vi "OFFSETEXPAND.vi"(9 "address string":string) -> ()   [LabVIEW 2013]
panel:
  out "data":string
  out "Expand":dbl format="%.2f"
  out "offset":dbl format="%.2f"
  out "data 2":string
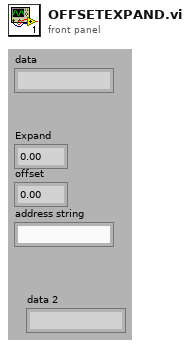
[diagram p1: front panel]
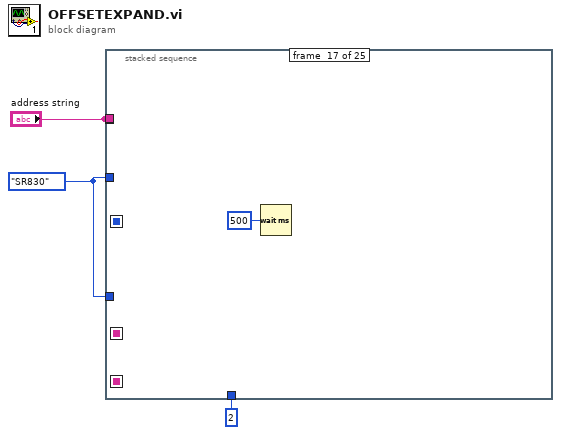
[diagram p0: block diagram]
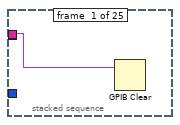
[diagram p2: hidden frame]
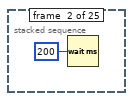
[diagram p3: hidden frame]
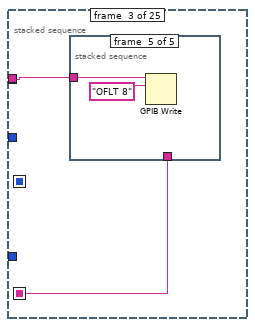
[diagram p4: hidden frame]
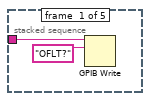
[diagram p5: hidden frame]
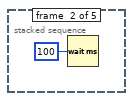
[diagram p6: hidden frame]
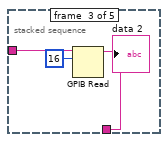
[diagram p7: hidden frame]
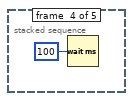
[diagram p8: hidden frame]
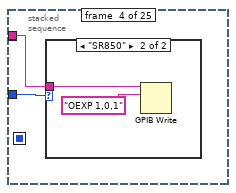
[diagram p9: hidden frame]
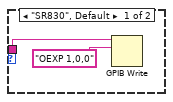
[diagram p10: hidden frame]
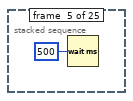
[diagram p11: hidden frame]
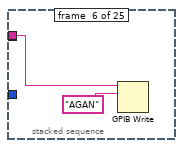
[diagram p12: hidden frame]
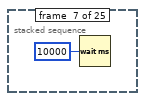
[diagram p13: hidden frame]
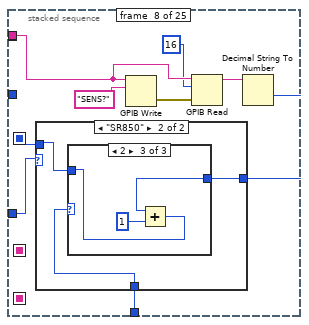
[diagram p14: hidden frame]
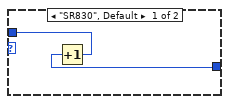
[diagram p15: hidden frame]
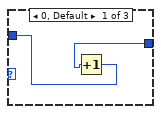
[diagram p16: hidden frame]
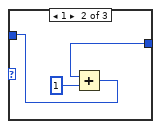
[diagram p17: hidden frame]
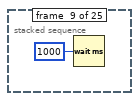
[diagram p18: hidden frame]
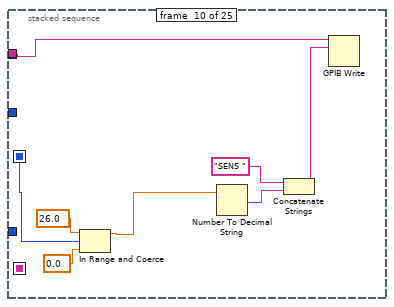
[diagram p19: hidden frame]
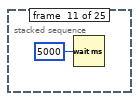
[diagram p20: hidden frame]
diagram:
  w2 = enum16{"SR830", "SR850"}."SR830" ("Lockin Type")
  n1 = stacked-sequence {
    seq-local: [_ _ _ _ _ _ _ _ _ _ _ _ _ _ _ _ _ w67 _ _ _ _ _ _ _] -> [_ _ _ _ _ _ _ _ _ _ _ _ _ _ _ _ _ _ _ w79 _ _ _ _ _]
    seq-local: [_ _ _ _ _ _ _ w29 _ _ _ _ _ _ _ _ _ _ _ _ _ _ _ _ _] -> [_ _ _ _ _ _ _ _ _ w51 _ _ _ _ _ _ _ _ _ _ _ _ _ _ _]
    seq-local: [_ _ w6 _ _ _ _ _ _ _ _ _ _ _ _ _ _ _ _ _ _ _ _ _ _] -> [_ _ _ _ _ _ _ _ _ _ _ _ _ _ _ _ _ _ _ _ _ _ _ w98 w104]
    tunnel: "address string" -> [w4 _ w7 _ _ _ _ w33 _ w57 _ w60 _ w62 _ w64 _ w72 _ w81 _ w94 _ w99 _]
    tunnel: "address string" -> [_ _ _ w18 _ w25 _ _ _ _ _ _ _ _ _ _ _ _ _ _ _ _ _ _ _]
    tunnel: w2 -> [_ _ _ _ _ _ _ w27 _ _ _ _ _ _ _ _ _ _ _ w76 _ _ _ _ _]
    tunnel: w2 -> [_ _ _ w17 _ _ _ _ _ _ _ _ _ _ _ _ _ _ _ _ _ _ _ _ _]
    tunnel: u16 2 ("Expand by") -> [_ _ _ _ _ _ _ w28 _ _ _ _ _ _ _ _ _ _ _ w75 _ _ _ _ _]
    frame #0 {
      n2 = GPIB Clear(3:w4) -> ()  [unwired: 1 in, 2 out]
    }
    frame #1 {
      n3 = Wait (ms)(milliseconds to wait=u32 200) -> ()  [unwired: 1 out]
    }
    frame #2 {
      n4 = stacked-sequence {
        tunnel: w7 -> [w9 _ w13 _ w16]
        tunnel: [_ _ w11 _ _] -> w6
        frame #0 {
          n5 = GPIB Write(0:w9, 1:"OFLT?" ("data")) -> ()  [unwired: 3 in, 2 out]
        }
        frame #1 {
          n6 = Wait (ms)(milliseconds to wait=u32 100) -> ()  [unwired: 1 out]
        }
        frame #2 {
          n7 = GPIB Read(0:w13, 1:16 ("byte count")) -> (5:w11:string)  [unwired: 3 in, 2 out]
          "data 2" <- w11
        }
        frame #3 {
          n8 = Wait (ms)(milliseconds to wait=u32 100) -> ()  [unwired: 1 out]
        }
        frame #4 {
          n9 = GPIB Write(0:w16, 1:"OFLT 8" ("data")) -> ()  [unwired: 3 in, 2 out]
        }
      }
    }
    frame #3 {
      n10 = case shown="\"SR850\"" w17 {
        tunnel: w18 -> [w19 w22]
        frame "SR830", Default {
          n11 = GPIB Write(0:w19, 1:"OEXP 1,0,0" ("data")) -> ()  [unwired: 3 in, 2 out]
        }
        frame "SR850" {
          n12 = GPIB Write(0:w22, 1:"OEXP 1,0,1" ("data")) -> ()  [unwired: 3 in, 2 out]
        }
      }
    }
    frame #4 {
      n13 = Wait (ms)(milliseconds to wait=u32 500) -> ()  [unwired: 1 out]
    }
    frame #5 {
      n14 = GPIB Write(0:w25, 1:"AGAN" ("data")) -> ()  [unwired: 3 in, 2 out]
    }
    frame #6 {
      n15 = Wait (ms)(milliseconds to wait=u32 10000) -> ()  [unwired: 1 out]
    }
    frame #7 {
      n16 = GPIB Write(0:w33, 1:"SENS?" ("data")) -> (6:w34:errorcluster)  [unwired: 3 in, 1 out]
      n17 = GPIB Read(0:w33, 1:16 ("byte count"), 3:w34) -> (5:w31:string)  [unwired: 2 in, 2 out]
      n18 = Decimal String To Number(string=w31) -> (number=w30:i32)  [unwired: 2 in, 1 out]
      n19 = case shown="\"SR850\"" w27 {
        tunnel: w30 -> [w37 w39]
        tunnel: [w36 w38] -> w29
        tunnel: w28 -> [_ w40]
        frame "SR830", Default {
          n20 = Increment(x=w37) -> (x+1=w36:i32)
        }
        frame "SR850" {
          n21 = case shown="2" w40 {
            tunnel: w39 -> [w42 w45 w48]
            tunnel: [w41 w43 w46] -> w38
            frame 0, Default {
              n22 = Increment(x=w42) -> (x+1=w41:i32)
            }
            frame 1 {
              n23 = Add(x=w45, y=1) -> (x+y=w43:i32)
            }
            frame 2 {
              n24 = Add(x=w48, y=1) -> (x+y=w46:i32)
            }
          }
        }
      }
    }
    frame #8 {
      n25 = Wait (ms)(milliseconds to wait=u32 1000) -> ()  [unwired: 1 out]
    }
    frame #9 {
      n26 = In Range and Coerce(upper limit=26.0, x=w51, lower limit=0.0) -> (coerced(x)=w50:dbl)  [unwired: 1 out]
      n27 = Number To Decimal String(number=w50) -> (decimal integer string=w56:string)  [unwired: 1 in]
      n28 = Concatenate Strings("SENS " ("string"), w56) -> (w54:string)
      n29 = GPIB Write(0:w57, 1:w54) -> ()  [unwired: 3 in, 2 out]
    }
    frame #10 {
      n30 = Wait (ms)(milliseconds to wait=u32 5000) -> ()  [unwired: 1 out]
    }
    frame #11 {
      n31 = GPIB Write(0:w60, 1:"AOFF 1" ("data")) -> ()  [unwired: 3 in, 2 out]
    }
    frame #12 {
      n32 = Wait (ms)(milliseconds to wait=u32 1000) -> ()  [unwired: 1 out]
    }
    frame #13 {
      n33 = GPIB Clear(3:w62) -> ()  [unwired: 1 in, 2 out]
    }
    frame #14 {
      n34 = Wait (ms)(milliseconds to wait=u32 500) -> ()  [unwired: 1 out]
    }
    frame #15 {
      n35 = GPIB Write(0:w64, 1:"OEXP? 1" ("data")) -> ()  [unwired: 3 in, 2 out]
    }
    frame #16 {
      n36 = Wait (ms)(milliseconds to wait=u32 500) -> ()  [unwired: 1 out]
    }
    frame #17 {
      n37 = GPIB Read(0:w72, 1:512 ("byte count")) -> (5:w69:string)  [unwired: 3 in, 2 out]
      "data" <- w69
      n38 = Scan From String(format string="%f,%d", input string=w69) -> (output 1=w68:dbl, output 2=→"Expand":dbl)  [unwired: 4 in, 3 out]
      "offset" <- w68
      n39 = Number To Fractional String(number=w68) -> (F-format string=w67:string)  [unwired: 3 in]
    }
    frame #18 {
      n40 = Wait (ms)(milliseconds to wait=u32 500) -> ()  [unwired: 1 out]
    }
    frame #19 {
      n41 = case shown="\"SR850\"" w76 {
        tunnel: w75 -> [w82 w88]
        tunnel: [w83 w87] -> w77
        frame "SR830", Default {
          n42 = case shown="2" w82 {
            tunnel: [",0" ("string") ",1" ("string") ",2" ("string")] -> w83
            frame 0, Default {
            }
            frame 1 {
            }
            frame 2 {
            }
          }
        }
        frame "SR850" {
          n43 = case shown="2" w88 {
            tunnel: [",1" ("string") ",10" ("string") ",100" ("string")] -> w87
            frame 0, Default {
            }
            frame 1 {
            }
            frame 2 {
            }
          }
        }
      }
      n44 = Concatenate Strings("OEXP 1," ("data"), w79, w77) -> (w78:string)
      n45 = GPIB Write(0:w81, 1:w78) -> ()  [unwired: 3 in, 2 out]
    }
    frame #20 {
      n46 = Wait (ms)(milliseconds to wait=u32 1000) -> ()  [unwired: 1 out]
    }
    frame #21 {
      n47 = GPIB Write(0:w94, 1:"AOFF 1" ("data")) -> ()  [unwired: 3 in, 2 out]
    }
    frame #22 {
      n48 = Wait (ms)(milliseconds to wait=u32 1000) -> ()  [unwired: 1 out]
    }
    frame #23 {
      n49 = Concatenate Strings("OFLT " ("data"), w98) -> (w96:string)
      n50 = GPIB Write(0:w99, 1:w96) -> ()  [unwired: 3 in, 2 out]
    }
    frame #24 {
      n51 = Decimal String To Number(string=w104) -> (number=w101:i32)  [unwired: 2 in, 1 out]
      n52 = case shown="19" w101 {
        tunnel: [1e-05 3e-05 0.0001 0.0003 0.001 0.003 0.01 0.03 0.1 0.3 1 3 10 30 100 300 1000 3000 10000 30000] -> w100
        frame 0, Default {
        }
        frame 1 {
        }
        frame 2 {
        }
        frame 3 {
        }
        frame 4 {
        }
        frame 5 {
        }
        frame 6 {
        }
        frame 7 {
        }
        frame 8 {
        }
        frame 9 {
        }
        frame 10 {
        }
        frame 11 {
        }
        frame 12 {
        }
        frame 13 {
        }
        frame 14 {
        }
        frame 15 {
        }
        frame 16 {
        }
        frame 17 {
        }
        frame 18 {
        }
        frame 19 {
        }
      }
      n53 = Multiply(x=w100, y=15000.0) -> (x*y=w102:dbl)
      n54 = Wait (ms)(milliseconds to wait=w102) -> ()  [unwired: 1 out]
    }
  }
